vi "TriggerMazeCam.vi"() -> ()   [LabVIEW 2021]
uses:
  <vilib>/DAQmx/write.llb/DAQmx Write (Digital Bool 1Line 1Point).vi
  <vilib>/DAQmx/create/channels.llb/DAQmx Create Channel (DO-Digital Output).vi
  <vilib>/DAQmx/miscellaneous.llb/DAQmx Fill In Error Info.vi
panel:
  in  "lines":tag
  in  "STOP  RECORDING":bool
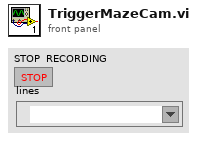
[diagram p1: front panel]
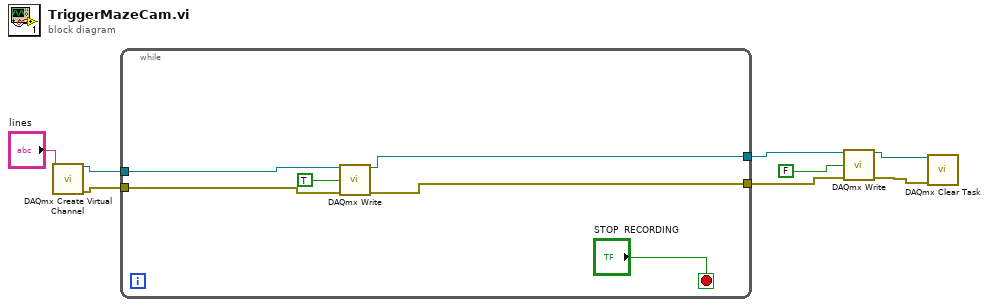
[diagram p0: block diagram]
diagram:
  n1 = call-poly <vilib>:"DAQmx Create Virtual Channel.vi"("lines"="lines") -> ("task out"=w8:refnum<k21>, "error out"=w7:errorcluster)  [unwired: 13 in]
  n2 = while {
    tunnel: w8 -> [w14]
    tunnel: w7 -> [w13]
    tunnel: [w10] -> w4
    tunnel: [w9] -> w3
    stop <- "STOP  RECORDING" stop-if-true
    n3 = call-poly <vilib>:"DAQmx Write.vi"("task/channels in"=w14, "data"=TRUE, "error in"=w13) -> ("task out"=w10:refnum<k21>, "error out"=w9:errorcluster)  [unwired: 10 in, 1 out]
  }
  n4 = call-poly <vilib>:"DAQmx Write.vi"("task/channels in"=w4, "data"=FALSE, "error in"=w3) -> ("task out"=w2:refnum<k21>, "error out"=w1:errorcluster)  [unwired: 10 in, 1 out]
  n5 = call <vilib>:"DAQmx Clear Task.vi"("task in"=w2, "error in"=w1) -> ()  [unwired: 13 in, 1 out]
